vi "add_info_from_text2.vi"(8 "error in (no error)":errorcluster, 10 "data array":string[](array[string]), 11 "AnalysisListItems in":refnum<class "AnalysisListItems.lvclass">) -> (0 "error out":errorcluster, 2 "data array out":string[](array[string]), 3 "AnalysisListItems out":refnum<class "AnalysisListItems.lvclass">)   [LabVIEW 2017, in "AnalysisListItems.lvclass"]
doc: "The VI seraches for keywords in the data array (lines of the data textfile) and adds the sample ifnormation in the AnalysisListItem Object.\n\nRunID\nAnalysisID\netc etc"
uses:
  AnalysisListItems.lvclass
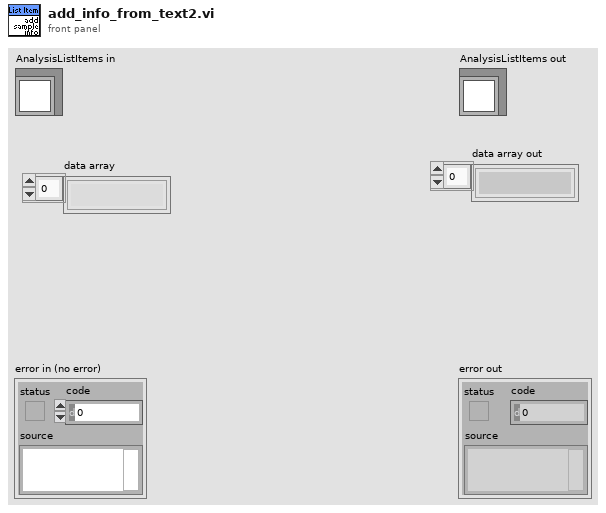
[diagram p1: front panel]
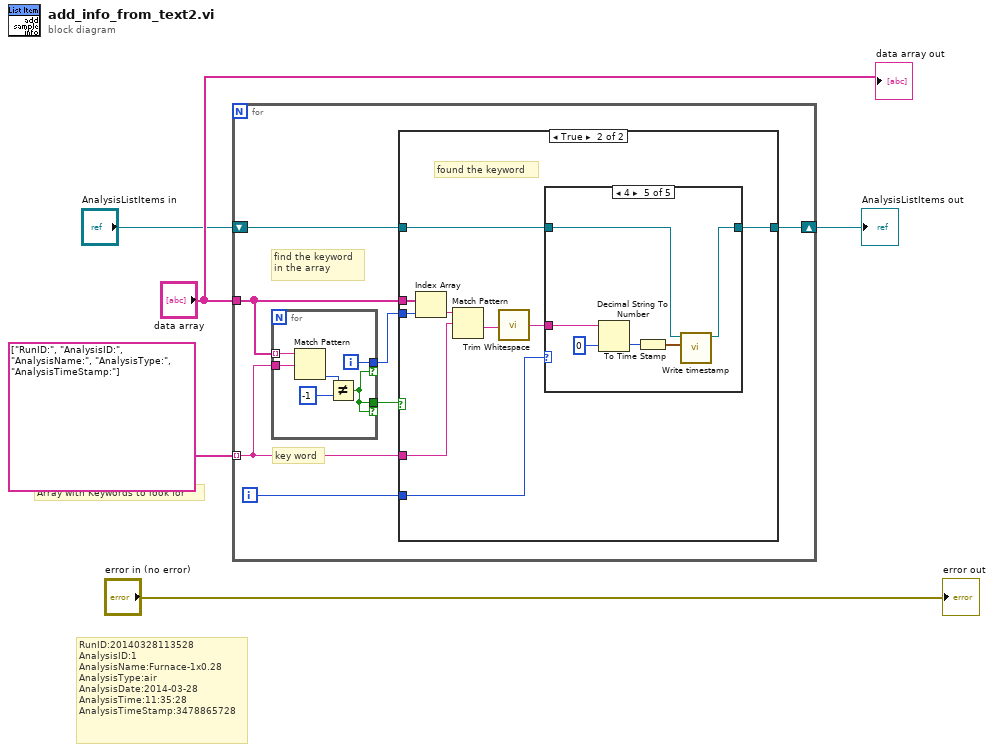
[diagram p0: block diagram]
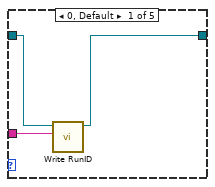
[diagram p3: hidden frame]
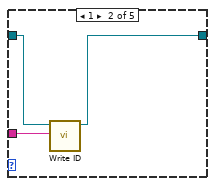
[diagram p4: hidden frame]
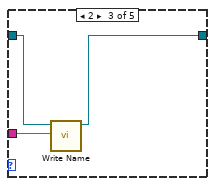
[diagram p5: hidden frame]
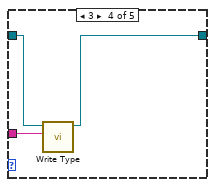
[diagram p6: hidden frame]
diagram:
  # "Array with Keywords to look for"
  # "RunID:20140328113528\nAnalysisID:1\nAnalysisName:Furnace-1x0.28\nAnalysisType:air\nAnalysisDate:2014-03-28\nAnalysisTime:11:35:28\nAnalysisTimeStamp:3478865728"
  n1 = for {
    tunnel: "data array" -> [w10]
    tunnel: string[] ["RunID:", "AnalysisID:", "AnalysisName:", "AnalysisType:", "AnalysisTimeStamp:"] -> [w9] mode=indexing
    shift-right: [w11] -> w1
    shift-left: "AnalysisListItems in" -> [w6]
    i -> [w12]
    # "find the keyword\nin the array"
    # "key word"
    n2 = for {
      tunnel: w10 -> [w46] mode=indexing
      tunnel: w9 -> [w45]
      tunnel: [w41] -> w8 if=w42
      tunnel: [w42] -> w7 if=w42
      i -> [w41]
      n3 = Match Pattern(string=w46, regular expression=w45) -> (offset past match=w44:i32)  [unwired: 1 in, 3 out]
      n4 = Not Equal?(x=w44, y=-1) -> (x != y?=w42:bool)
    }
    n5 = case shown="True" w7 {
      tunnel: w12 -> [_ w21]
      tunnel: w6 -> [w13 w18]
      tunnel: [w13 w17] -> w11
      tunnel: w10 -> [_ w16]
      tunnel: w9 -> [_ w15]
      tunnel: w8 -> [_ w14]
      frame False {
        # "didn' find the keyword"
      }
      frame True {
        # "found the keyword"
        n6 = Index Array(array=w16, index=w14) -> (element=w22:string)
        n7 = Match Pattern(string=w22, regular expression=w15) -> (after substring=w20:string)  [unwired: 1 in, 3 out]
        n8 = call <vilib>:"Trim Whitespace.vi"("string"=w20) -> ("trimmed string"=w19:string)  [unwired: 1 in]
        n9 = case shown="4" w21 {
          tunnel: w19 -> [w25 w28 w31 w34 w40]
          tunnel: [w23 w26 w29 w32 w36] -> w17
          tunnel: w18 -> [w24 w27 w30 w33 w35]
          frame 0, Default {
            n10 = call-dynamic "Write RunID.vi"("RunID"=w25, "AnalysisListItems in"=w24) -> ("AnalysisListItems out"=w23:refnum<class "AnalysisListItems.lvclass">)  [unwired: 8 in, 1 out]
          }
          frame 1 {
            n11 = call-dynamic "Write ID.vi"("ID"=w28, "AnalysisListItems in"=w27) -> ("AnalysisListItems out"=w26:refnum<class "AnalysisListItems.lvclass">)  [unwired: 8 in, 1 out]
          }
          frame 2 {
            n12 = call-dynamic "Write Name.vi"("Name"=w31, "AnalysisListItems in"=w30) -> ("AnalysisListItems out"=w29:refnum<class "AnalysisListItems.lvclass">)  [unwired: 8 in, 1 out]
          }
          frame 3 {
            n13 = call-dynamic "Write Type.vi"("Type"=w34, "AnalysisListItems in"=w33) -> ("AnalysisListItems out"=w32:refnum<class "AnalysisListItems.lvclass">)  [unwired: 8 in, 1 out]
          }
          frame 4 {
            n14 = Decimal String To Number(string=w40, default (0L)=i64 0) -> (number=w39:i64)  [unwired: 1 in, 1 out]
            n15 = To Time Stamp(1:w39) -> (0:w38:timestamp)
            n16 = call-dynamic "Write timestamp.vi"("timestamp"=w38, "AnalysisListItems in"=w35) -> ("AnalysisListItems out"=w36:refnum<class "AnalysisListItems.lvclass">)  [unwired: 8 in, 1 out]
          }
        }
      }
    }
  }
  "AnalysisListItems out" <- w1
  "error out" <- "error in (no error)"
  "data array out" <- "data array"
